vi "Read Benchmarks.vi"(11 "CIFChannels in":refnum<class "CIFChannels.lvclass">) -> (2 "Flatten (us)":T1, 3 "Channel R/W (us)":T1)   [LabVIEW 2021, in "CIFChannels.lvclass"]
uses:
  CIFChannels.lvclass
  <vilib>/CIF Foundation/CIF Utilities/Statistics/I64/Stats_I64_CIF_U.lvclass
  ChannelCommon/typedef/Benchmark Stats.ctl
  ChannelCommon/ChannelCommon.lvlib
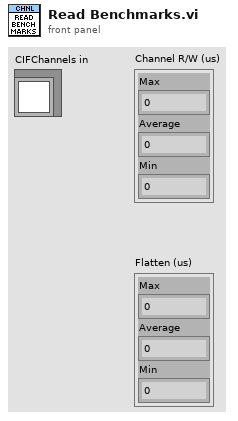
[diagram p1: front panel]
types:
  T1 = typedef "ChannelCommon.lvlib/Benchmark Stats.ctl" = cluster{"Max":i64, "Average":dbl, "Min":i64}
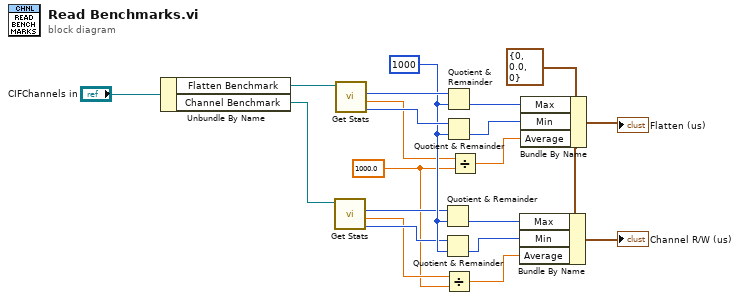
[diagram p0: block diagram]
diagram:
  w1 = T1 {"Max"=0, "Average"=0.0, "Min"=0} ("Flatten (us)")
  w10 = 1000.0 ("y")
  w15 = i64 1000 ("y")
  n1 = Unbundle By Name("CIFChannels in") -> ("Flatten Benchmark"=w18:refnum<class "Stats_I64_CIF_U.lvclass">, "Channel Benchmark"=w19:refnum<class "Stats_I64_CIF_U.lvclass">)
  n2 = call <vilib>:"Get Stats.vi"("Stats_I64_CIF_U in"=w19) -> ("Min"=w13:i64, "Average"=w11:dbl, "Max"=w14:i64)  [unwired: 6 in, 2 out]
  n3 = call <vilib>:"Get Stats.vi"("Stats_I64_CIF_U in"=w18) -> ("Min"=w16:i64, "Average"=w12:dbl, "Max"=w17:i64)  [unwired: 6 in, 2 out]
  n4 = Quotient & Remainder(x=w14, y=w15) -> (floor(x/y)=w6:i64)  [unwired: 1 out]
  n5 = Quotient & Remainder(x=w13, y=w15) -> (floor(x/y)=w5:i64)  [unwired: 1 out]
  n6 = Quotient & Remainder(x=w17, y=w15) -> (floor(x/y)=w9:i64)  [unwired: 1 out]
  n7 = Quotient & Remainder(x=w16, y=w15) -> (floor(x/y)=w8:i64)  [unwired: 1 out]
  n8 = Divide(x=w11, y=w10) -> (x/y=w4:dbl)
  n9 = Divide(x=w12, y=w10) -> (x/y=w7:dbl)
  n10 = Bundle By Name(cluster=w1, "Max"=w6, "Min"=w5, "Average"=w4) -> (→"Channel R/W (us)":T1)
  n11 = Bundle By Name(cluster=w1, "Max"=w9, "Min"=w8, "Average"=w7) -> (→"Flatten (us)":T1)
